vi "niFpgaDcRmsOutsideSCTLWindow.vi"(0 "input data":fxp<+/-,32,1>, 1 "reset":bool) -> (2 "Sum result":fxp<+/-,42,11> format="%.35g", 4 "DC result":fxp<+/-,32,1> format="%.32g", 6 "RMS result":fxp<+,32,1> format="%.32g", 8 "Mean Square result":fxp<+,63,1> format="%.63g", 10 "results valid":bool)   [LabVIEW 2017]
doc: "Calculates the <B>DC (Mean)</B> and/or <B>RMS</B> values of an input signal. You also can use this VI to calculate the intermediate <B>Sum</B>, <B>Mean Square</B>, and <B>Square Sum</B> values in order to save FPGA resources."
uses:
  <vilib>/rvi/FXPMathLib/basic elements/FxpIntAccumulator/XNode/nifxpmath_IntAccumulator.xnode
  <vilib>/rvi/FXPMathLib/basic elements/FxpIntAccumulator/simVIs/DllFxpIntAccumulator_sub.vi
  <vilib>/rvi/FXPMathLib/basic elements/FxpIntAccumulator/subVIs/nifxpmath_IntAccumulator_SimConfig.ctl
  <vilib>/rvi/FXPMathLib/FxpMul/XNode/nifxpmath_Multiplier.xnode
  <vilib>/fxp/LVFixedPointOverflowPolicyTypeDef.ctl
  <vilib>/rvi/FXPMathLib/FxpSqrt/XNode/nifxpmath_Sqrt.xnode
  <vilib>/Platform/TimedLoop/XDataNode/XDataNode.xnode
  <vilib>/Platform/TimedLoop/XDataNode/nitl_modes.ctl
  <vilib>/Platform/TimedLoop/XDataNode/XDNodeRunTimeDep.lvlib
  <vilib>/Platform/TimedLoop/XDataNode/wakeup.ctl
  <vilib>/Platform/TimedLoop/XDataNode/timing_clust.ctl
  <vilib>/rvi/FXPMathLib/FxpSqrt/simVIs/DllSqrtTemp_sub.vi
  <vilib>/rvi/FXPMathLib/FxpSqrt/subVIs/nifxpmath_Sqrt_SimConfig.ctl
  <vilib>/rvi/FXPMathLib/sim/FxpSim.dll
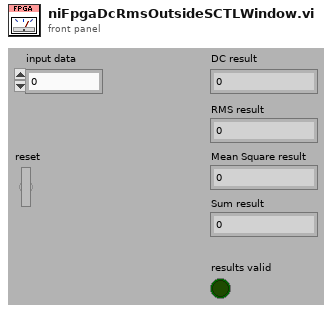
[diagram p1: front panel]
types:
  T1 = typedef "XDNodeRunTimeDep.lvlib/timing_clust.ctl" = cluster{"Expected End [f-1]":u64, "Actual End [f-1]":u64, "Finished Late? [f-1]":bool, "Expected End [i-1]":u64, "Actual End [i-1]":u64, "Finished Late? [i-1]":bool, "Expected Start [i]":u64, "Actual Start [i]":u64, "Expected Start [f]":u64, "Actual Start [f]":u64, "Source Name":string, "Structure Name":string, "Period":i64, "Deadline":i64, "Offset":i64, "Start":i64, "Priority":i32, "Timeout":i32, "Mode":T2, "Wakeup Reason":T3, "Error":errorcluster, "Source Type":string, "Secondary Source Type":string, "Global End Time":u64, "Global Start Time":u64, "Frame Duration":u64, "Iteration Duration":u64, "Assigned CPU":i32, "I/O Scan Engine Mode":u32}
  T2 = typedef "XDNodeRunTimeDep.lvlib/nitl_modes.ctl" = enum32{"No Change", "Process missed periods, maintain original phase", "Discard missed periods, maintain original phase", "Process missed periods, ignore original phase", "Discard missed periods, ignore original phase"}
  T3 = typedef "XDNodeRunTimeDep.lvlib/wakeup.ctl" = enum32{"Normal", "Aborted", "Asynchronous wakeup", "Timing source error", "Timed loop error", "Timeout"}
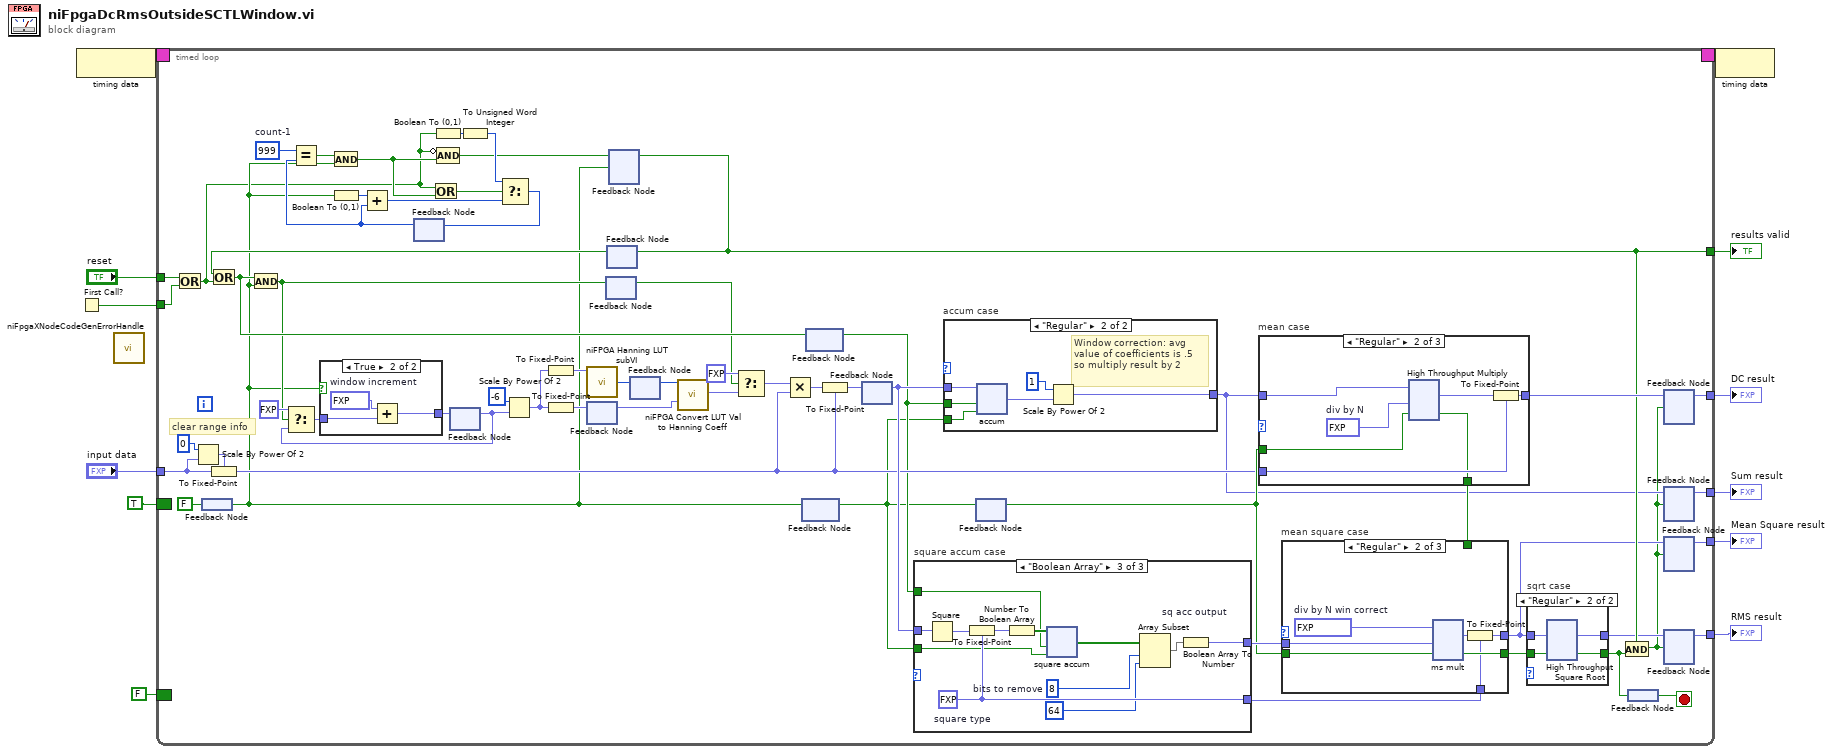
[diagram p0: block diagram]
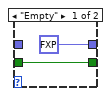
[diagram p3: hidden frame]
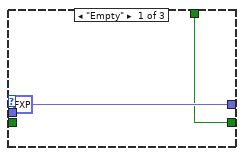
[diagram p4: hidden frame]
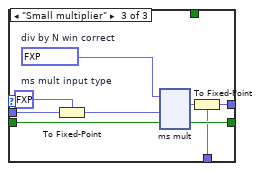
[diagram p5: hidden frame]
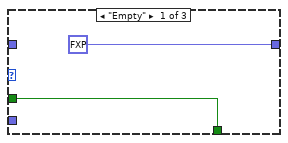
[diagram p6: hidden frame]
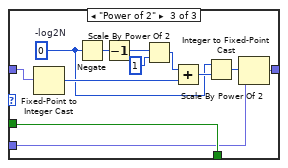
[diagram p7: hidden frame]
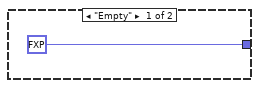
[diagram p8: hidden frame]
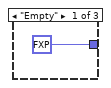
[diagram p9: hidden frame]
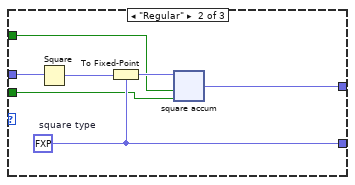
[diagram p10: hidden frame]
diagram:
  n1 = node-c288() -> (w10:T1)
  n2 = First Call?() -> (First Call?: T/F=w11:bool)
  n3 = call <vilib>:"niFpgaXNodeCodeGenErrorHandle.vi"() -> ()  [unwired: 1 in]
  n4 = timed-loop {
    tunnel: [w15] -> w4
    tunnel: "input data" -> [w32]
    tunnel: "reset" -> [w68]
    tunnel: w11 -> [w67]
    tunnel: [w18] -> w2
    tunnel: [w20] -> w1
    tunnel: [w23] -> w8
    tunnel: [w16] -> w3
    timing: w10 -> [_]
    timing-out: [_] -> w9
    border: TRUE -> [_]
    border: FALSE -> [_]
    stop <- w24 stop-if-true
    w72 = u16 999  # count-1
    # "clear range info"
    n5 = Or(x=w68, y=w67) -> (x .or. y?=w13:bool)
    n6 = Scale By Power Of 2(n=0, x=w32) -> (x*2^n=w34:fxp<+/-,32,1>)
    n7 = feedback #1() -> (w26:bool)
    n8 = feedback-in #1(FALSE) -> ()
    n9 = To Fixed-Point(fixed-point type=w34, number=w32) -> (fixed-point=w31:fxp<+/-,32,1>)
    n10 = Boolean To (0,1)(Boolean=w26) -> (0, 1=w66:i16)
    n11 = feedback #2() -> (w60:u16)  [unwired: 1 in]
    n12 = Equal?(x=w72, y=w60) -> (x = y?=w64:bool)
    n13 = And(x=w64, y=w26) -> (x .and. y?=w62:bool)
    n14 = Add(x=w66, y=w60) -> (x+y=w65:u16)
    n15 = Or(x=w13, y=w62) -> (x .or. y?=w63:bool)
    n16 = Boolean To (0,1)(Boolean=w13) -> (0, 1=w71:i16)
    n17 = Compound Arithmetic op=AND(invert w13, w62) -> (w57:bool)
    n18 = feedback #3() -> (w48:fxp<+,32,16>)  [unwired: 1 in]
    n19 = To Unsigned Word Integer(number=w71) -> (unsigned 16bit integer=w70:u16)
    n20 = Select(t=w70, s=w63, f=w65) -> (s? t:f=w69:u16)
    n21 = feedback-in #2(w69) -> ()
    n22 = Scale By Power Of 2(n=-6, x=w48) -> (x*2^n=w46:fxp<+,32,16>)
    n23 = To Fixed-Point(number=w46) -> (fixed-point=w38:fxp<+,10,10>)  [unwired: 1 in]
    n24 = To Fixed-Point(number=w46) -> (fixed-point=w47:fxp<+,16,0>)  [unwired: 1 in]
    n25 = call <vilib>:"niFPGA Hanning LUT subVI.vi"("address"=w38) -> ("data out"=w37:u32)  [unwired: 7 in]
    n26 = feedback-in #4(w47) -> ()
    n27 = feedback #4() -> (w52:fxp<+,16,0>)  [unwired: 1 in]
    n28 = feedback #5() -> (w43:bool)  [unwired: 1 in]
    n29 = feedback #6() -> (w61:bool)  [unwired: 1 in]
    n30 = Or(x=w61, y=w13) -> (x .or. y?=w44:bool)
    n31 = And(x=w44, y=w26) -> (x .and. y?=w29:bool)
    n32 = Select(t=fxp<+,32,16> 0.0, s=w29, f=w48) -> (s? t:f=w55:fxp<+,32,16>)
    n33 = case shown="True" w26 {
      tunnel: [w73 w76] -> w42
      tunnel: w55 -> [w73 w74]
      frame False {
      }
      frame True {
        w75 = fxp<+,32,16> 65.53599548339844  # window increment
        n34 = Add(x=w75, y=w74) -> (x+y=w76:fxp<+,32,16>)
      }
    }
    n35 = feedback-in #3(w42) -> ()
    n36 = feedback-in #5(w29) -> ()
    n37 = feedback-in #7(w57, w26) -> ()
    n38 = feedback #7() -> (w23:bool)  [unwired: 1 in]
    n39 = feedback-in #6(w23) -> ()
    n40 = feedback-in #8(w37) -> ()
    n41 = feedback #8() -> (w41:u32)  [unwired: 1 in]
    n42 = call <vilib>:"niFPGA Convert LUT Val to Hanning Coeff.vi"("LUT value"=w41, "fractional index"=w52) -> ("Hanning coefficient"=w53:fxp<+,17,0>)  [unwired: 13 in]
    n43 = Select(t=fxp<+,17,0> 0.0 ("Hanning (U16)"), s=w43, f=w53) -> (s? t:f=w50:fxp<+,17,0>)
    n44 = Multiply(x=w50, y=w31) -> (x*y=w54:fxp<+/-,49,1>)
    n45 = feedback #9() -> (w25:bool)  [unwired: 1 in]
    n46 = feedback-in #9(w26) -> ()
    n47 = feedback-in #10(w44) -> ()
    n48 = feedback #10() -> (w27:bool)  [unwired: 1 in]
    n49 = To Fixed-Point(fixed-point type=w31, number=w54) -> (fixed-point=w36:fxp<+/-,32,1>)
    n50 = feedback-in #11(w36) -> ()
    n51 = feedback #11() -> (w35:fxp<+/-,32,1>)  [unwired: 1 in]
    n52 = case "square accum case" shown="\"Boolean Array\"" {
      selector: _ -> [_ _ _]
      tunnel: w35 -> [_ w185 w225]
      tunnel: w25 -> [_ w182 w216]
      tunnel: w27 -> [_ w181 w215]
      tunnel: [fxp<+,1,1> 0.0 ("s") w184 w217] -> w56
      tunnel: [_ w183 w224] -> w58
      frame "Empty" {
      }
      frame "Regular" {
        w183 = fxp<+,63,1> 0.0  # square type
        n53 = Square(x=w185) -> (x^2=w187:fxp<+,63,1>)
        n54 = To Fixed-Point(fixed-point type=w183, number=w187) -> (fixed-point=w186:fxp<+,63,1>)
        n55 = xnode "square accum"("x"=w186, "load (F)"=w181, "enable (T)"=w182) -> ("s"=w184:fxp<+,63,1>)  [unwired: 2 in, 1 out]
      }
      frame "Boolean Array" {
        w221 = 8  # bits to remove
        w224 = fxp<+,63,1> 0.0  # square type
        n56 = Square(x=w225) -> (x^2=w226:fxp<+,63,1>)
        n57 = To Fixed-Point(fixed-point type=w224, number=w226) -> (fixed-point=w223:fxp<+,63,1>)
        n58 = Number To Boolean Array(number=w223) -> (Boolean array=w222:bool[])
        n59 = xnode "square accum"("x"=w222, "load (F)"=w215, "enable (T)"=w216) -> ("s"=w218:bool[])  [unwired: 2 in, 1 out]
        n60 = Array Subset(array=w218, index=w221, length=64) -> (w219:bool[])
        n61 = Boolean Array To Number "sq acc output"(Boolean array=w219) -> (number=w217:fxp<+,64,10>)
      }
    }
    n62 = case "accum case" shown="\"Regular\"" {
      selector: _ -> [_ _]
      tunnel: w35 -> [_ w152]
      tunnel: w25 -> [_ w151]
      tunnel: w27 -> [_ w150]
      tunnel: [fxp<+/-,42,11> 0.0 ("input data") w147] -> w17
      frame "Empty" {
      }
      frame "Regular" {
        # "Window correction: avg value of coefficients is .5 so multiply result by 2"
        n63 = xnode "accum"("x"=w152, "load (F)"=w150, "enable (T)"=w151) -> ("s"=w148:fxp<+/-,49,18>)  [unwired: 2 in, 1 out]
        n64 = Scale By Power Of 2(n=1, x=w148) -> (x*2^n=w147:fxp<+/-,49,18>)
      }
    }
    n65 = feedback-in #12(w25) -> ()
    n66 = feedback #12() -> (w40:bool)  [unwired: 1 in]
    n67 = case "mean case" shown="\"Regular\"" {
      selector: _ -> [_ _ _]
      tunnel: [fxp<+/-,32,1> 0.0 ("input data") w133 w134] -> w28
      tunnel: w17 -> [_ w131 w136]
      tunnel: w31 -> [_ w130 w135]
      tunnel: w40 -> [w126 w129 w145]
      tunnel: [w126 w127 w145] -> w39
      frame "Empty" {
      }
      frame "Regular" {
        w128 = fxp<+,17,-9> 0.0010000020265579224  # div by N
        n68 = xnode "High Throughput Multiply"("x"=w131, "y"=w128, "input valid"=w129) -> ("x*y"=w132:fxp<+/-,64,9>, "output valid"=w127:bool)  [unwired: 1 in, 1 out]
        n69 = To Fixed-Point(fixed-point type=w130, number=w132) -> (fixed-point=w133:fxp<+/-,32,1>)
      }
      frame "Power of 2" {
        w137 = i8 0  # -log2N
        n70 = Fixed-Point to Integer Cast(1:w136) -> (0:w140:i64)
        n71 = Negate(x=w137) -> (-x=w144:i8)
        n72 = Decrement(x=w144) -> (x-1=w143:i8)
        n73 = Scale By Power Of 2(n=w143, x=i64 1 ("x-1")) -> (x*2^n=w141:i64)
        n74 = Add(x=w141, y=w140) -> (x+y=w138:i64)
        n75 = Scale By Power Of 2(n=w137, x=w138) -> (x*2^n=w139:i64)
        n76 = Integer to Fixed-Point Cast(fixed-point type=w135, integer=w139) -> (fixed-point=w134:fxp<+/-,32,1>)
      }
    }
    n77 = case "mean square case" shown="\"Regular\"" {
      selector: _ -> [_ _ _]
      tunnel: [w107 w115 w124] -> w59
      tunnel: [fxp<+,63,1> 0.0 ("input data") w113 w122] -> w19
      tunnel: w58 -> [_ w112 w121]
      tunnel: w56 -> [_ w111 w120]
      tunnel: w40 -> [_ w109 w117]
      tunnel: w39 -> [w107 _ _]
      frame "Empty" {
      }
      frame "Regular" {
        w110 = fxp<+,17,-8> 0.0026667118072509766  # div by N win correct
        n78 = xnode ("ms mult")("x"=w110, "y"=w111, "input valid"=w109) -> ("x*y"=w114:fxp<+,64,2>, "output valid"=w115:bool)  [unwired: 1 in, 1 out]
        n79 = To Fixed-Point(fixed-point type=w112, number=w114) -> (fixed-point=w113:fxp<+,63,1>)
      }
      frame "Small multiplier" {
        w116 = fxp<+,17,-8> 0.002666652202606201  # div by N win correct
        w118 = fxp<+,34,10> 0.0  # ms mult input type
        n80 = To Fixed-Point(fixed-point type=w118, number=w120) -> (fixed-point=w119:fxp<+,34,10>)
        n81 = xnode ("ms mult")("x"=w116, "y"=w119, "input valid"=w117) -> ("x*y"=w123:fxp<+,51,2>, "output valid"=w124:bool)  [unwired: 1 in, 1 out]
        n82 = To Fixed-Point(fixed-point type=w121, number=w123) -> (fixed-point=w122:fxp<+,63,1>)
      }
    }
    n83 = case "sqrt case" shown="\"Regular\"" {
      selector: _ -> [_ _]
      tunnel: [fxp<+,32,1> 0.0 ("input data") w82] -> w21
      tunnel: [w78 w81] -> w22
      tunnel: w59 -> [w78 w80]
      tunnel: w19 -> [_ w79]
      frame "Empty" {
      }
      frame "Regular" {
        n84 = xnode "High Throughput Square Root"("x"=w79, "input valid"=w80) -> ("sqrt(x)"=w82:fxp<+,32,1>, "output valid"=w81:bool)  [unwired: 1 in, 1 out]
      }
    }
    n85 = And(x=w23, y=w22) -> (x .and. y?=w14:bool)
    n86 = feedback #13() -> (w24:bool)
    n87 = feedback-in #13(w22) -> ()
    n88 = feedback #14() -> (w15:fxp<+/-,32,1>)  [unwired: 1 in]
    n89 = feedback-in #14(w28, w14) -> ()
    n90 = feedback #15() -> (w16:fxp<+/-,49,18>)  [unwired: 1 in]
    n91 = feedback-in #15(w17, w14) -> ()
    n92 = feedback #16() -> (w18:fxp<+,63,1>)  [unwired: 1 in]
    n93 = feedback-in #16(w19, w14) -> ()
    n94 = feedback #17() -> (w20:fxp<+,32,1>)  [unwired: 1 in]
    n95 = feedback-in #17(w21, w14) -> ()
  }
  "results valid" <- w8
  "DC result" <- w4
  "Mean Square result" <- w2
  "RMS result" <- w1
  "Sum result" <- w3
  n96 = node-c288(w9) -> ()
